vi "Match.vi"(1 "SSNFromProduct":string, 2 "RescannedSSN":string) -> (0 "x = y?":bool)   [LabVIEW 2014]
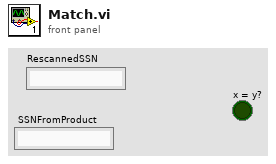
[diagram p1: front panel]
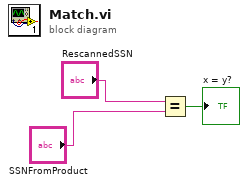
[diagram p0: block diagram]
diagram:
  n1 = Equal?(x="RescannedSSN", y="SSNFromProduct") -> (x = y?=→"x = y?":bool)
